vi "Write Channel State.vi"(8 "error in (no error)":errorcluster, 10 "State":T1, 11 "Channel in":refnum<data-value>) -> (0 "error out":errorcluster, 3 "Channel out":refnum<data-value>)   [LabVIEW 2020, in "G-Audio.lvlib" / "Channel.lvclass"]
uses:
  Channel.lvclass
  Channel State.ctl
  Channel.lvclass/Channel.ctl
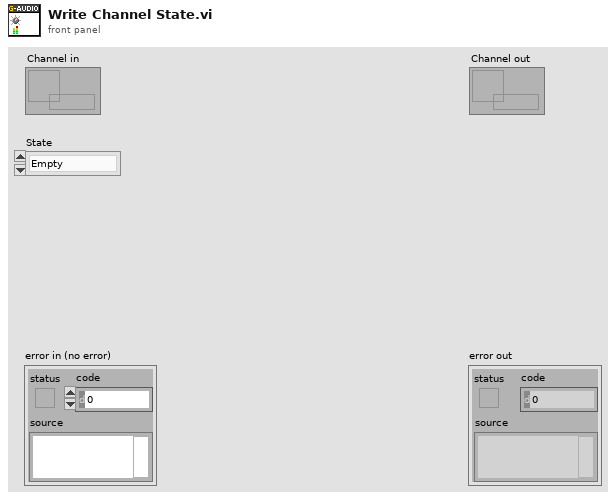
[diagram p1: front panel]
types:
  T1 = typedef "G-Audio.lvlib/Channel.lvclass/Channel State.ctl" = enum16{"Empty", "Loading", "Stopped", "Paused", "Playing", "Retrigger"}
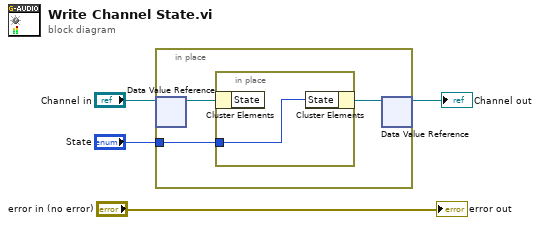
[diagram p0: block diagram]
diagram:
  n1 = in-place {
    in-place-border: "State" -> [w6]
    n2 = in-place-dvr #1("Channel in") -> (w7:refnum<class "Channel.lvclass">)  [unwired: 1 out]
    n3 = in-place {
      in-place-border: w6 -> [w8]
      n4 = in-place-cluster #2(w7) -> ()  [unwired: 1 out]
      n5 = in-place-cluster #2("State"=w8) -> (w5:refnum<class "Channel.lvclass">)
    }
    n6 = in-place-dvr #1(w5) -> (→"Channel out":refnum<data-value>)  [unwired: 1 out]
  }
  "error out" <- "error in (no error)"
